vi "Port.vi"() -> ()   [LabVIEW 2023]
panel:
  in  "Cluster":T1
  out "Available (mB)":i64
  in  "Transfer (mB)":i64
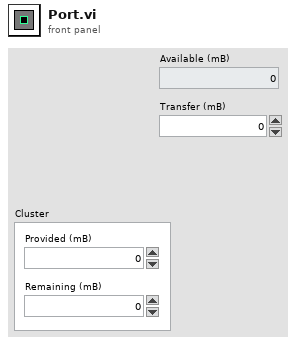
[diagram p1: front panel]
types:
  T1 = cluster{"Remaining (mB)":i64, "Provided (mB)":i64}
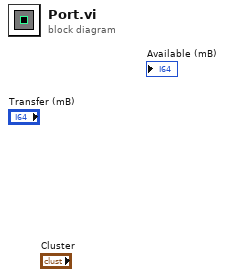
[diagram p0: block diagram]
diagram:
